vi "Save.vi"(8 "error in":errorcluster, 10 "file path":path, 11 "repository in":refnum<class "modification container.lvclass">) -> (0 "error out":errorcluster, 3 "repository out":refnum<class "modification container.lvclass">)   [LabVIEW 2013, in "modification container.lvclass"]
doc: "Stores repo information to file. It could save in multiple files or formats at the same time. File versioning is suggested."
uses:
  modification container.lvclass
  modification container.lvclass/modification container.ctl
  FileCluster.ctl
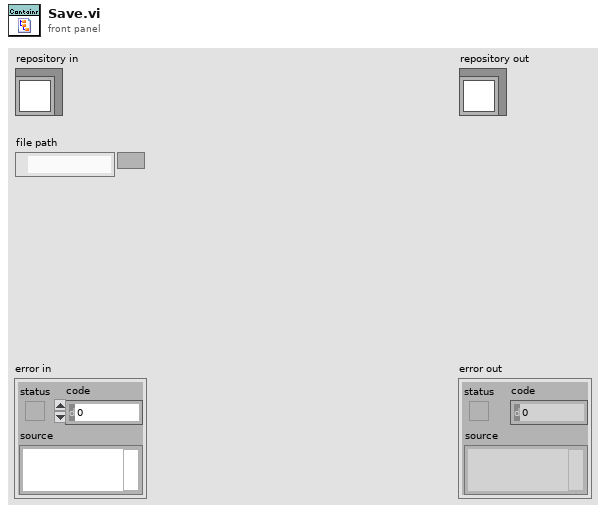
[diagram p1: front panel]
types:
  T1 = typedef "modification container.lvclass/FileCluster.ctl" = cluster{"Version":string, "Data":variant}
  T2 = enum16{"open", "replace", "create", "open or create", "replace or create", "replace or create with confirmation"}
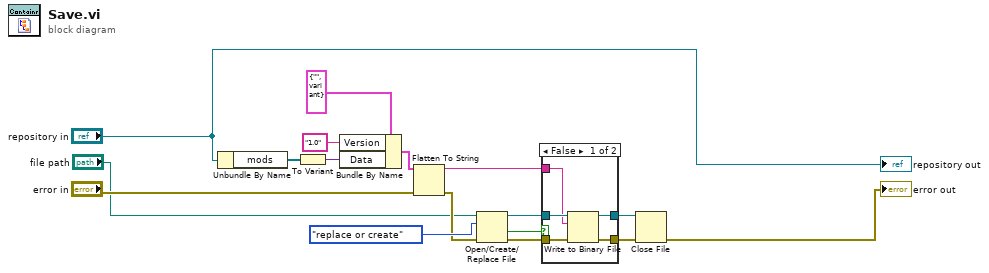
[diagram p0: block diagram]
diagram:
  n1 = Unbundle By Name("repository in") -> ("mods"=w16:refnum<class "VI modification.lvclass">[])
  n2 = To Variant(anything=w16) -> (Variant=w17:variant)
  n3 = Bundle By Name(cluster=T1 {"Version"="", "Data"=variant}, "Version"="1.0" ("Version String"), "Data"=w17) -> (w7:T1)
  n4 = Flatten To String(anything=w7, error in (no error)="error in") -> (data string=w6:string, error out=w5:errorcluster)  [unwired: 2 in, 1 out]
  n5 = Open/Create/Replace File(file path (use dialog)="file path", error in=w5, operation (0:open)=T2."replace or create") -> (refnum out=w9:refnum<file>, cancelled=w12:bool, error out=w13:errorcluster)  [unwired: 3 in]
  n6 = case shown="False" w12 {
    tunnel: w13 -> [w22 w23]
    tunnel: [w21 w23] -> w11
    tunnel: [w20 w24] -> w10
    tunnel: w9 -> [w19 w24]
    tunnel: w6 -> [w18 _]
    frame False {
      n7 = Write to Binary File(file (use dialog)=w19, data=w18, error in=w22) -> (refnum out=w20:refnum<file>, error out=w21:errorcluster)  [unwired: 3 in, 1 out]
    }
    frame True {
    }
  }
  n8 = Close File(refnum=w10, error in=w11) -> (error out=→"error out":errorcluster)  [unwired: 1 out]
  "repository out" <- "repository in"
